vi "FTW-XML-Query-Elements.vi"(0 "XML Node":refnum<k20>, 5 "XPath Query":string, 11 "error in":errorcluster) -> (4 "XML Node out":refnum<k20>, 6 "Matching Nodes":refnum<k20>[](array[refnum]), 8 "Num Matches":i32, 15 "error out":errorcluster)   [LabVIEW 2015]
uses:
  error/FTW-ERR-CallChain.vi
  error/FTW-ERR-NoErrorConstant.vi
  string/FTW-STR-ReplaceWhitespace.vi
  string/FTW-STR-Array-Delimit.vi
  error/FTW-ERR-Clear.vi
  regex/FTW-Regex-ReplaceAll.vi
  DOMUserDefRef.dll
panel:
  # "Inputs"
  # "Outputs"
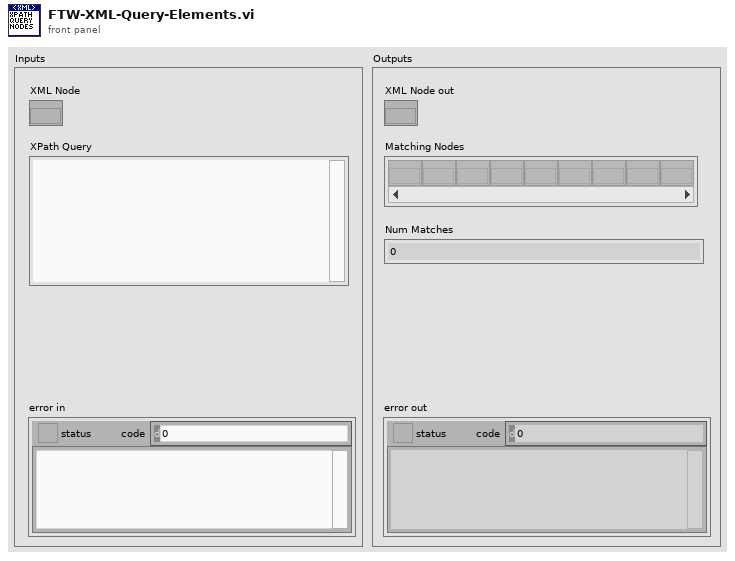
[diagram p1: front panel]
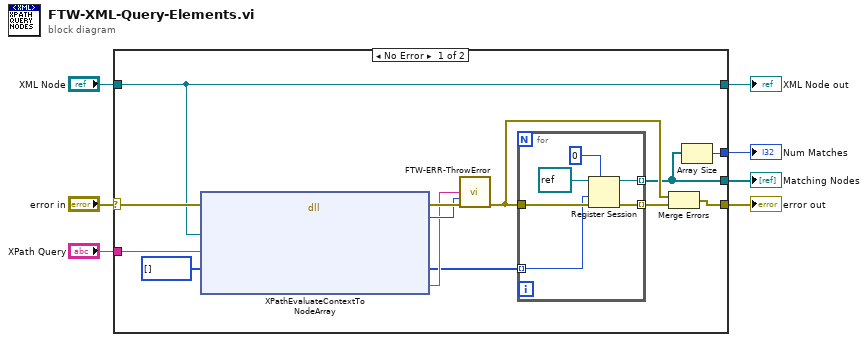
[diagram p0: block diagram]
diagram:
  n1 = case shown="No Error" "error in" {
    selector: "error in" -> [w20 w28]
    tunnel: [w11 w28] -> w7
    tunnel: "XML Node" -> [w17 w27]
    tunnel: [w17 w27] -> w4
    tunnel: "XPath Query" -> [w18 _]
    tunnel: [w10 _] -> w2
    tunnel: [w9 _] -> w1
    frame No Error {
      n2 = dll-call lib="DOMUserDefRef.*" fn="XPathEvaluateContextToNodeArray"(error in=w20, "Base Node"=w17, "XPath Query"=w18, "Matching Nodes"=u64[] []) -> (error out=w19:errorcluster, "Return"=w16:i32, "Matching Nodes"=w14:u64[], "Error String"=w15:string)  [unwired: 3 in, 3 out]
      n3 = call "FTW-ERR-ThrowError.vi"("Error Message"=w15, "Error Code"=w16, "error in"=w19) -> ("error out"=w13:errorcluster)  [unwired: 12 in]
      n4 = for {
        tunnel: w13 -> [w24]
        tunnel: [w23] -> w10 mode=indexing
        tunnel: w14 -> [w22] mode=indexing
        tunnel: [w21] -> w12 mode=indexing
        n5 = Register Session(7:0 ("cleanup mode (default to class = 0)"), 8:w24, 9:w22, 11:refnum<k20> refnum ("refnum")) -> (0:w21:errorcluster, 3:w23:refnum<k20>)  [unwired: 1 in]
      }
      n6 = Merge Errors(w13, w12) -> (w11:errorcluster)
      n7 = Array Size(array=w10) -> (size(s)=w9:i32)
    }
    frame Error {
    }
  }
  "error out" <- w7
  "XML Node out" <- w4
  "Matching Nodes" <- w2
  "Num Matches" <- w1
